vi "Login Request.vi"(8 "error in (no error)":errorcluster, 9 "password":string, 10 "username":string, 11 "[C] User Management in":refnum<class "[C] User Management.lvclass">) -> (0 "error out":errorcluster, 3 "[C] User Management out":refnum<class "[C] User Management.lvclass">)   [LabVIEW 2020, in "[C] User Management.lvlib" / "[C] User Management.lvclass"]
uses:
  [C] User Management.lvclass
  [C] User Management.lvclass/[C] User Management.ctl
  <vilib>/ActorFramework/Message Enqueuer/Message Enqueuer.lvclass/Message Enqueuer.ctl
  <vilib>/ActorFramework/Message Enqueuer/Enqueue.vi
  [V] Login/[V] Login Messages/Login Fail Msg/Login Fail Msg.lvclass
  C:/Program Files (x86)/National Instruments/LabVIEW 2020/vi.lib/ActorFramework/Message/Message.lvclass
  <vilib>/ActorFramework/Stop Msg/Stop Msg.lvclass
  <vilib>/ActorFramework/Message Priority Queue/Priority Enqueue.vi
  [Data] Userinfo/[Data] Abstruct Userinfo/[Data] Abstruct Userinfo.lvclass
  [Data] Recent User/[Data] Recent User.lvclass
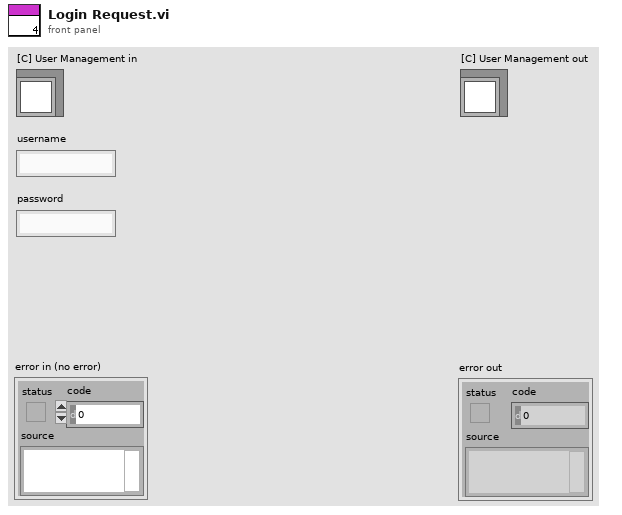
[diagram p1: front panel]
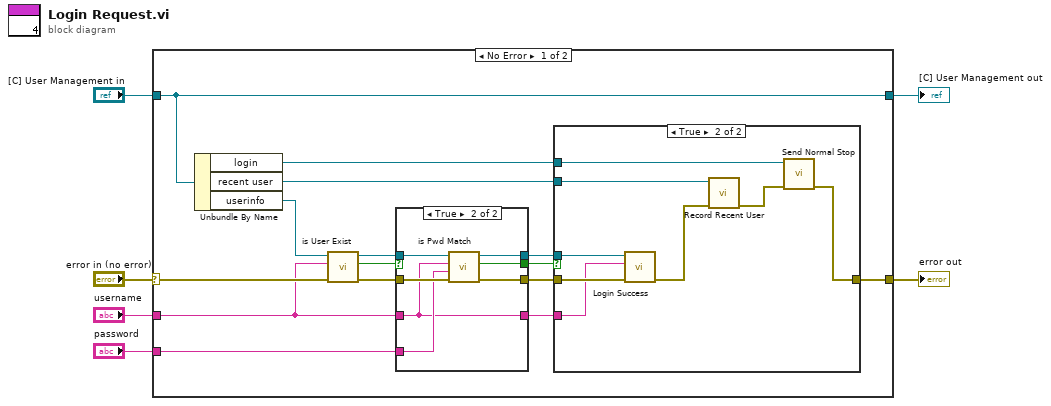
[diagram p0: block diagram]
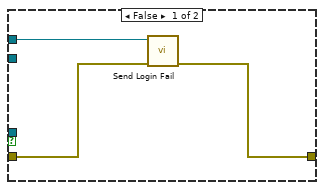
[diagram p2: hidden frame]
diagram:
  n1 = case shown="No Error" "error in (no error)" {
    selector: "error in (no error)" -> [w21 w45]
    tunnel: [w11 w45] -> w4
    tunnel: "[C] User Management in" -> [w8 w44]
    tunnel: [w8 w44] -> w3
    tunnel: "username" -> [w15 _]
    tunnel: "password" -> [w16 _]
    frame No Error {
      n2 = Unbundle By Name(w8) -> ("login"=w9:refnum<class "Message Enqueuer.lvclass">, "recent user"=w7:refnum<class "[Data] Recent User.lvclass">, "userinfo"=w20:refnum<class "[Data] Abstruct Userinfo.lvclass">)
      n3 = call-dynamic "is User Exist.vi"("error in (no error)"=w21, "username"=w15, "[Data] Abstruct Userinfo in"=w20) -> ("error out"=w19:errorcluster, "exist?"=w18:bool, "[Data] Abstruct Userinfo out"=w17:refnum<class "[Data] Abstruct Userinfo.lvclass">)  [unwired: 6 in]
      n4 = case shown="True" w18 {
        selector: w18 -> [w34 _]
        tunnel: w19 -> [w35 w42]
        tunnel: w17 -> [w36 w43]
        tunnel: [w36 w40] -> w12
        tunnel: [w35 w39] -> w14
        tunnel: w16 -> [_ w41]
        tunnel: w15 -> [w33 w37]
        tunnel: [w34 w38] -> w13
        tunnel: [w33 w37] -> w10
        frame False {
        }
        frame True {
          n5 = call-dynamic "is Pwd Match.vi"("error in (no error)"=w42, "password"=w41, "username"=w37, "[Data] Abstruct Userinfo in"=w43) -> ("error out"=w39:errorcluster, "match?"=w38:bool, "[Data] Abstruct Userinfo out"=w40:refnum<class "[Data] Abstruct Userinfo.lvclass">)  [unwired: 5 in]
        }
      }
      n6 = case shown="True" w13 {
        tunnel: w14 -> [w24 w32]
        tunnel: w12 -> [_ w31]
        tunnel: [w22 w28] -> w11
        tunnel: w10 -> [_ w30]
        tunnel: w9 -> [w23 w29]
        tunnel: w7 -> [_ w27]
        frame False {
          n7 = call "Send Login Fail.vi"("error in (no error)"=w24, "Message Enqueuer"=w23) -> ("error out"=w22:errorcluster)  [unwired: 8 in, 1 out]
        }
        frame True {
          n8 = call-dynamic "Login Success.vi"("error in (no error)"=w32, "username"=w30, "[Data] Abstruct Userinfo in"=w31) -> ("error out"=w26:errorcluster)  [unwired: 7 in, 1 out]
          n9 = call "Record Recent User.vi"("error in (no error)"=w26, "[Data] Recent User in"=w27) -> ("error out"=w25:errorcluster)  [unwired: 8 in, 1 out]
          n10 = call <vilib>:"Send Normal Stop.vi"("error in (no error)"=w25, "Message Enqueuer"=w29) -> ("error out"=w28:errorcluster)  [unwired: 9 in]
        }
      }
    }
    frame Error {
    }
  }
  "error out" <- w4
  "[C] User Management out" <- w3
